vi "attributes2Variant.vi"(0 "HGF_PVBase":refnum<class "HGF_PVBase.lvclass">, 2 "Parameter":variant, 3 "typeDescriptor":string, 5 "error in (no error)":errorcluster) -> (14 "HGF_PVBase":refnum<class "HGF_PVBase.lvclass">, 16 "rawData":variant, 19 "error out":errorcluster)   [LabVIEW 2014, in "HGF_BaseClasses.lvlib" / "HGF_PVBase.lvclass"]
doc: "Convert variant attributes Pn, n=0,1,2,... to raw data value of variant."
uses:
  HGF_PVBase.lvclass
  HGF_PVDataConverter/HGF_PVDataConverter.lvclass
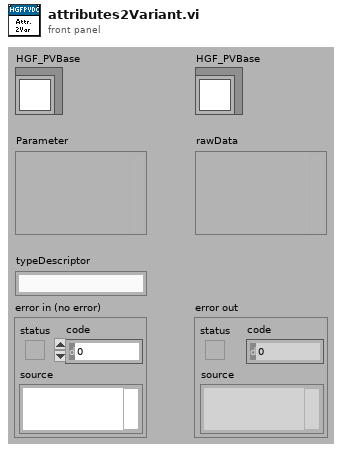
[diagram p1: front panel]
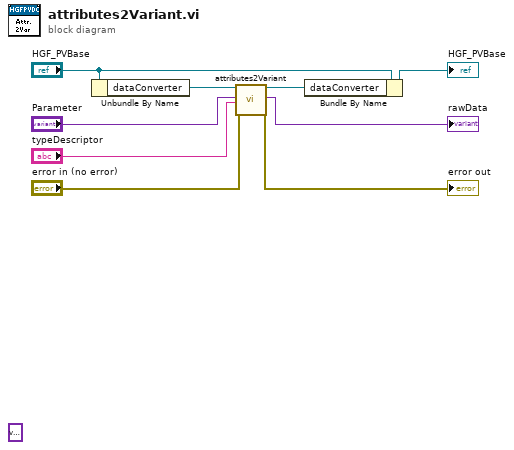
[diagram p0: block diagram]
diagram:
  (unwired) variant ("rawData")
  (unwired) variant ("rawData")
  n1 = Unbundle By Name("HGF_PVBase") -> ("dataConverter"=w7:refnum<class "HGF_PVDataConverter.lvclass">)
  n2 = call-dynamic "attributes2Variant.vi"("HGF_PVDataConverter"=w7, "Parameter"="Parameter", "typeDescriptor"="typeDescriptor", "error in (no error)"="error in (no error)") -> ("HGF_PVDataConverter"=w6:refnum<class "HGF_PVDataConverter.lvclass">, "rawData"=→"rawData":variant, "error out"=→"error out":errorcluster)  [unwired: 13 out]
  n3 = Bundle By Name(cluster="HGF_PVBase", "dataConverter"=w6) -> (→"HGF_PVBase":refnum<class "HGF_PVBase.lvclass">)
